vi "Initialize.vi"(8 "error in (no error)":errorcluster, 9 "Default remote state (Local)":u16(ring) items=["Local", "Remote"], 10 "Reset (True)":bool=TRUE, 11 "VISA resource name":refnum<visa-resource-name>) -> (0 "error out":errorcluster, 3 "VISA resource name out":refnum<visa-resource-name>)   [LabVIEW 2020, in "Datron D4xxx.lvlib"]
doc: "Establishes communication with the instrument and optionally performs an instrument identification query and/or an instrument reset. It also places the instrument in a default state needed for other instrument driver operations. Therefore, call this VI before calling other instrument driver VIs for this instrument. Generally, you need to call the Initialize VI only once at the beginning of an application."
uses:
  Datron D4xxx.lvlib
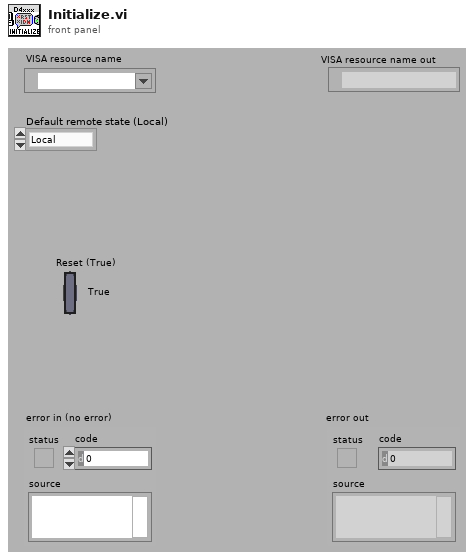
[diagram p1: front panel]
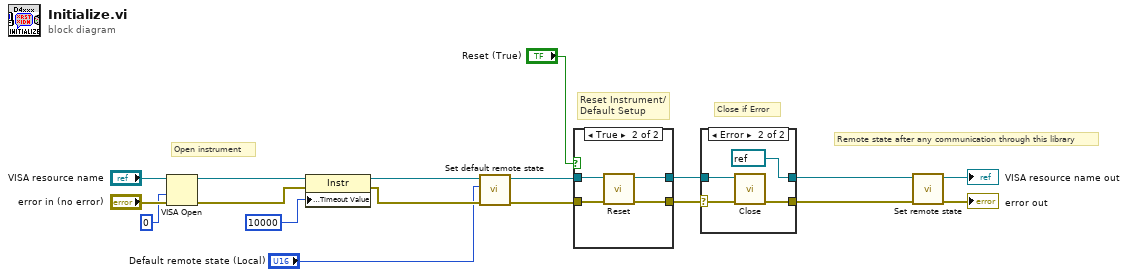
[diagram p0: block diagram]
diagram:
  # "Remote state after any communication through this library"
  # "Close if Error"
  # "Reset Instrument/\nDefault Setup"
  # "Open instrument"
  n1 = VISA Open(access mode=u32 0, error in (no error)="error in (no error)", VISA resource name="VISA resource name") -> (VISA resource name=w10:refnum<visa-resource-name>, error out=w11:errorcluster)  [unwired: 2 in]
  n2 = property class="Instr"(reference=w10, error in=w11, "General Settings:Timeout Value"=u32 10000) -> (reference out=w5:refnum<visa-resource-name>, error out=w4:errorcluster)
  n3 = call "Set default remote state.vi"("error in (no error)"=w4, "Default remote state (Local)"="Default remote state (Local)", "VISA resource name"=w5) -> ("error out"=w7:errorcluster, "VISA resource name out"=w6:refnum<visa-resource-name>)  [unwired: 7 in]
  n4 = case shown="True" "Reset (True)" {
    tunnel: w7 -> [w19 w21]
    tunnel: [w19 w24] -> w12
    tunnel: w6 -> [w20 w22]
    tunnel: [w20 w23] -> w13
    frame False {
    }
    frame True {
      n5 = call "Reset.vi"("error in (no error)"=w21, "VISA resource name"=w22) -> ("error out"=w24:errorcluster, "VISA resource name out"=w23:refnum<visa-resource-name>)  [unwired: 8 in]
    }
  }
  n6 = case shown="Error" w12 {
    selector: w12 -> [w25 w28]
    tunnel: w13 -> [w26 w29]
    tunnel: [w26 refnum<visa-resource-name> refnum ("VISA resource name out")] -> w2
    tunnel: [w25 w30] -> w1
    frame No Error {
    }
    frame Error {
      n7 = call "Close.vi"("error in (no error)"=w28, "VISA resource name"=w29) -> ("error out"=w30:errorcluster)  [unwired: 9 in]
    }
  }
  n8 = call "Set remote state.vi"("error in"=w1, "VISA resource name"=w2) -> ("error out"=→"error out":errorcluster, "VISA resource name out"=→"VISA resource name out":refnum<visa-resource-name>)  [unwired: 8 in]
